vi "StopStage.vi"(8 "error in":errorcluster, 11 "reference in":refnum<k7>) -> (0 "error out":errorcluster, 2 "result string":string, 3 "reference out":refnum<k7>)   [LabVIEW 2020]
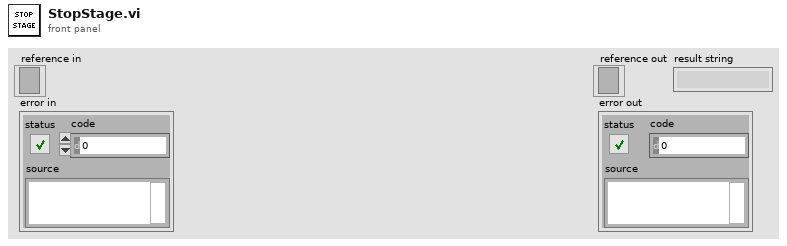
[diagram p1: front panel]
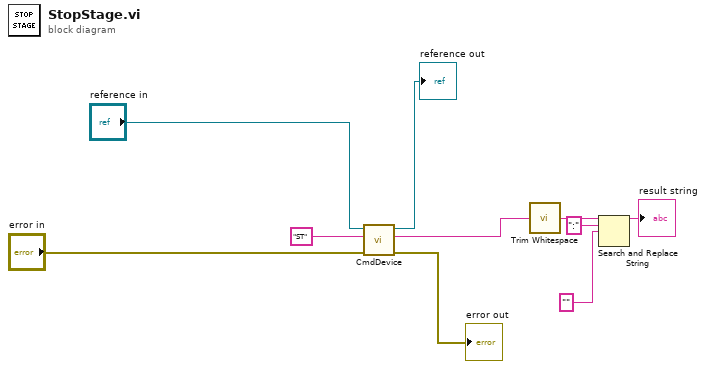
[diagram p0: block diagram]
diagram:
  n1 = call "CmdDevice.vi"("error in (no error)"="error in", "Command:"="ST" ("format string"), "reference in"="reference in") -> ("error out"=→"error out":errorcluster, "Response:"=w4:string, "reference out"=→"reference out":refnum<k7>)  [unwired: 6 in]
  n2 = call <vilib>:"Trim Whitespace.vi"("string"=w4) -> ("trimmed string"=w7:string)  [unwired: 1 in]
  n3 = Search and Replace String(input string=w7, search string=":", replace string="" ("replace string (\"\")")) -> (result string=→"result string":string)  [unwired: 5 in, 3 out]
